vi "Jason Recursion Binary Tube Search SubVI.vi"(6 "Beginning Tube Number":i32, 7 "End Tube Number":i32, 8 "Clear Pin Task In":refnum<k21>, 9 "Write Pin Task In":refnum<k21>, 10 "Sync Pin Task In":refnum<k21>, 11 "Data Pin Task In":refnum<k21>) -> (0 "Clear Pin Task Out":refnum<k21>, 1 "Write Pin Task Out":refnum<k21>, 2 "Sync Pin Task Out":refnum<k21>, 3 "Data Pin Task Out":refnum<k21>)   [LabVIEW 2020]
uses:
  <vilib>/numeric/Random Number (Range) DBL.vi
panel:
  out "Sync Pin Task Out 3":refnum<k21>[](array[refnum])
  out "Write Pin Task Out 3":refnum<k21>[](array[refnum])
  out "Data Pin Task Out 3":refnum<k21>[](array[refnum])
  out "Clear Pin Task Out 3":refnum<k21>[](array[refnum])
  out "Sync Pin Task Out 2":refnum<k21>[](array[refnum])
  out "Write Pin Task Out 2":refnum<k21>[](array[refnum])
  out "Data Pin Task Out 2":refnum<k21>[](array[refnum])
  out "Clear Pin Task Out 2":refnum<k21>[](array[refnum])
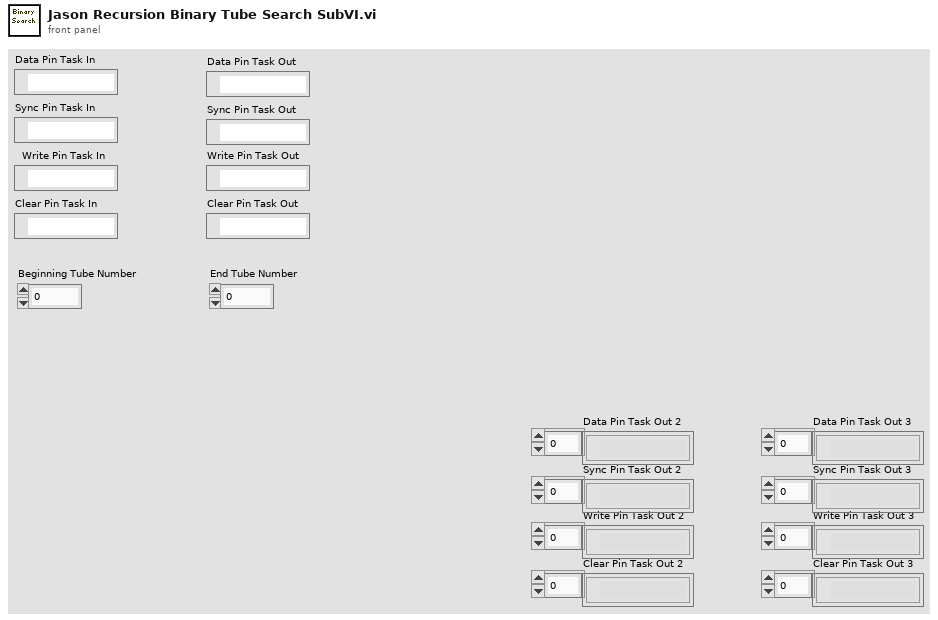
[diagram p1: front panel]
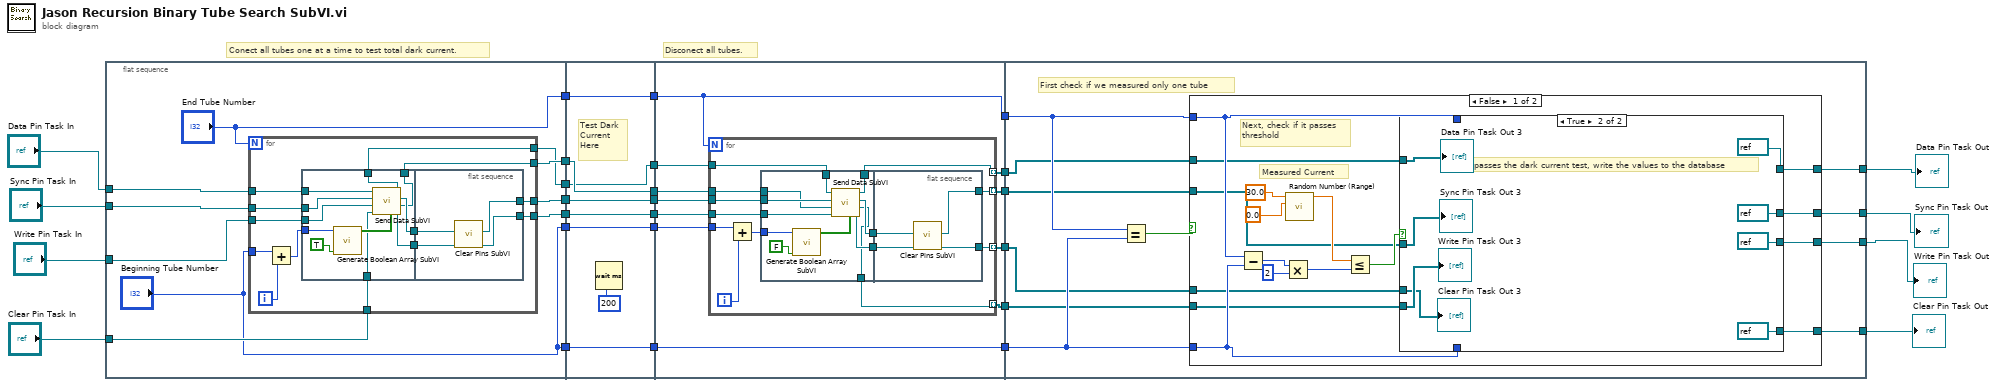
[diagram p0: block diagram]
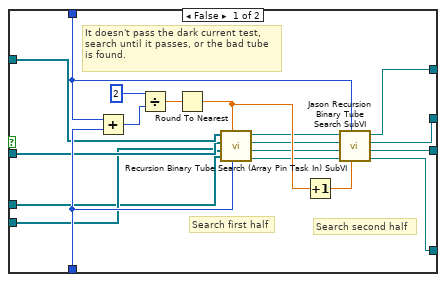
[diagram p2: hidden frame]
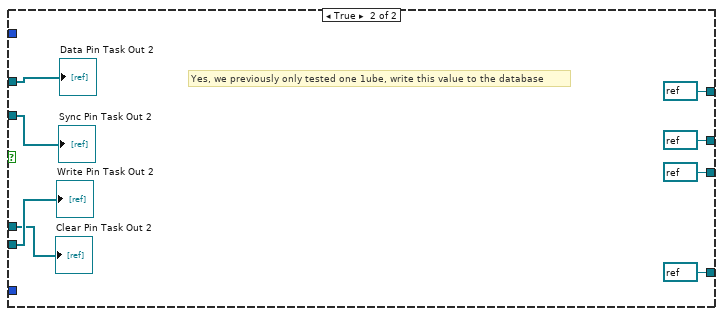
[diagram p3: hidden frame]
diagram:
  # "Disconect all tubes."
  # "Conect all tubes one at a time to test total dark current."
  n1 = flat-sequence {
    tunnel: "Data Pin Task In" -> [w38]
    tunnel: "Sync Pin Task In" -> [w37]
    tunnel: "Write Pin Task In" -> [w36]
    tunnel: "Clear Pin Task In" -> [w35]
    tunnel: ["End Tube Number"] -> w23
    tunnel: [w33] -> w21
    tunnel: [w32] -> w19
    tunnel: [w31] -> w17
    tunnel: [w30] -> w15
    tunnel: ["Beginning Tube Number"] -> w12
    tunnel: ["Beginning Tube Number"] -> w9
    tunnel: [w73] -> w24
    tunnel: w23 -> [w73]
    tunnel: [w72] -> w22
    tunnel: w21 -> [w72]
    tunnel: [w71] -> w20
    tunnel: w19 -> [w71]
    tunnel: [w70] -> w18
    tunnel: w17 -> [w70]
    tunnel: [w69] -> w16
    tunnel: w15 -> [w69]
    tunnel: [w68] -> w13
    tunnel: w12 -> [w68]
    tunnel: [w67] -> w10
    tunnel: w9 -> [w67]
    tunnel: w24 -> [w81]
    tunnel: w22 -> [w85]
    tunnel: w20 -> [w84]
    tunnel: w18 -> [w83]
    tunnel: w16 -> [w82]
    tunnel: [w81] -> w14
    tunnel: w13 -> [w80]
    tunnel: [w79] -> w11
    tunnel: w10 -> [w79]
    tunnel: [w78] -> w8
    tunnel: [w77] -> w7
    tunnel: [w76] -> w6
    tunnel: [w75] -> w5
    tunnel: w14 -> [w123]
    tunnel: w11 -> [w122]
    tunnel: w8 -> [w117]
    tunnel: w7 -> [w116]
    tunnel: w6 -> [w115]
    tunnel: w5 -> [w114]
    tunnel: [w121] -> w4
    tunnel: [w120] -> w3
    tunnel: [w119] -> w2
    tunnel: [w118] -> w1
    frame #0 {
      n2 = for {
        N: "End Tube Number" -> [_]
        tunnel: w38 -> [w51]
        tunnel: w37 -> [w50]
        tunnel: w36 -> [w49]
        tunnel: w35 -> [w48]
        tunnel: [w45] -> w33
        tunnel: [w44] -> w32
        tunnel: [w43] -> w31
        tunnel: [w42] -> w30
        tunnel: "Beginning Tube Number" -> [w39]
        i -> [w40]
        n3 = Add(x=w39, y=w40) -> (x+y=w41:i32)
        n4 = flat-sequence {
          tunnel: w41 -> [w60]
          tunnel: w51 -> [w59]
          tunnel: w50 -> [w58]
          tunnel: w49 -> [w57]
          tunnel: w48 -> [w56]
          tunnel: [w55] -> w47
          tunnel: [w54] -> w46
          tunnel: [w53] -> w43
          tunnel: [w52] -> w42
          tunnel: w47 -> [w66]
          tunnel: w46 -> [w65]
          tunnel: [w64] -> w45
          tunnel: [w63] -> w44
          frame #0 {
            n5 = call "Generate Boolean Array SubVI.vi"("Activate: 1\nDeactivate: 0"=TRUE, "Tube"=w60) -> ("Boolean array"=w61:bool[])  [unwired: 9 in]
            n6 = call "Send Data SubVI.vi"("Data Pin Task In"=w59, "Sync Pin Task In"=w58, "Write Pin Task In"=w57, "Clear Pin Task In"=w56, "Data"=w61) -> ("Data Pin Task Out"=w52:refnum<k21>, "Sync Pin Task Out"=w55:refnum<k21>, "Write Pin Task Out"=w53:refnum<k21>, "Clear Pin Task Out"=w54:refnum<k21>)  [unwired: 1 in]
          }
          frame #1 {
            n7 = call "Clear Pins SubVI.vi"("Clear Pin Task In"=w65, "Sync Pin Task In"=w66) -> ("Clear Pin Task Out"=w63:refnum<k21>, "Sync Pin Task Out"=w64:refnum<k21>)  [unwired: 8 in]
          }
        }
      }
    }
    frame #1 {
      # "Test Dark \nCurrent \nHere"
      n8 = Wait (ms)(milliseconds to wait=u32 200) -> ()  [unwired: 1 out]
    }
    frame #2 {
      n9 = for {
        N: w81 -> [_]
        tunnel: w85 -> [w96]
        tunnel: w84 -> [w95]
        tunnel: w83 -> [w94]
        tunnel: w82 -> [w93]
        tunnel: w80 -> [w90]
        tunnel: [w89] -> w78 mode=indexing
        tunnel: [w88] -> w77 mode=indexing
        tunnel: [w87] -> w76 mode=indexing
        tunnel: [w86] -> w75 mode=indexing
        i -> [w91]
        n10 = Add(x=w90, y=w91) -> (x+y=w92:i32)
        n11 = flat-sequence {
          tunnel: w92 -> [w107]
          tunnel: [w106] -> w98
          tunnel: [w105] -> w97
          tunnel: w96 -> [w104]
          tunnel: w95 -> [w103]
          tunnel: w94 -> [w102]
          tunnel: w93 -> [w101]
          tunnel: [w100] -> w89
          tunnel: [w99] -> w87
          tunnel: w98 -> [w113]
          tunnel: w97 -> [w112]
          tunnel: [w111] -> w88
          tunnel: [w110] -> w86
          frame #0 {
            n12 = call "Generate Boolean Array SubVI.vi"("Activate: 1\nDeactivate: 0"=FALSE, "Tube"=w107) -> ("Boolean array"=w108:bool[])  [unwired: 9 in]
            n13 = call "Send Data SubVI.vi"("Data Pin Task In"=w101, "Sync Pin Task In"=w104, "Write Pin Task In"=w102, "Clear Pin Task In"=w103, "Data"=w108) -> ("Data Pin Task Out"=w100:refnum<k21>, "Sync Pin Task Out"=w106:refnum<k21>, "Write Pin Task Out"=w99:refnum<k21>, "Clear Pin Task Out"=w105:refnum<k21>)  [unwired: 1 in]
          }
          frame #1 {
            n14 = call "Clear Pins SubVI.vi"("Clear Pin Task In"=w112, "Sync Pin Task In"=w113) -> ("Clear Pin Task Out"=w110:refnum<k21>, "Sync Pin Task Out"=w111:refnum<k21>)  [unwired: 8 in]
          }
        }
      }
    }
    frame #3 {
      # "First check if we measured only one tube"
      n15 = Equal?(x=w123, y=w122) -> (x = y?=w124:bool)
      n16 = case shown="False" w124 {
        tunnel: w123 -> [w134 _]
        tunnel: w122 -> [w133 _]
        tunnel: [w132 refnum<k21> refnum ("Data Pin Task Out")] -> w121
        tunnel: [w131 refnum<k21> refnum ("Sync Pin Task Out")] -> w120
        tunnel: [w130 refnum<k21> refnum ("Write Pin Task Out")] -> w119
        tunnel: [w129 refnum<k21> refnum ("Clear Pin Task Out")] -> w118
        tunnel: w117 -> [w128 w172]
        tunnel: w116 -> [w127 w171]
        tunnel: w115 -> [w126 w170]
        tunnel: w114 -> [w125 w169]
        frame False {
          # "Next, check if it passes\nthreshold"
          # "Measured Current"
          n17 = Subtract(x=w134, y=w133) -> (x-y=w136:i32)
          n18 = Multiply(x=w136, y=2) -> (x*y=w141:i32)
          n19 = call-poly <vilib>:"Random Number (Range).vi"("lower bound (0)"=0.0, "upper bound (100)"=30.0) -> ("number"=w140:dbl)  [unwired: 9 in]
          n20 = Less Or Equal?(x=w140, y=w141) -> (x <= y?=w135:bool)
          n21 = case shown="True" w135 {
            tunnel: w134 -> [w157 _]
            tunnel: w133 -> [w150 _]
            tunnel: [w155 refnum<k21> refnum ("Data Pin Task Out")] -> w132
            tunnel: [w154 refnum<k21> refnum ("Sync Pin Task Out")] -> w131
            tunnel: [w153 refnum<k21> refnum ("Write Pin Task Out")] -> w130
            tunnel: [w152 refnum<k21> refnum ("Clear Pin Task Out")] -> w129
            tunnel: w128 -> [w145 w168]
            tunnel: w127 -> [w144 w167]
            tunnel: w126 -> [w143 w166]
            tunnel: w125 -> [w142 w165]
            frame False {
              # "Search second half"
              # "Search first half"
              # "It doesn't pass the dark current test,\nsearch until it passes, or the bad tube\nis found."
              n22 = Add(x=w157, y=w150) -> (x+y=w159:i32)
              n23 = Divide(x=2, y=w159) -> (x/y=w160:dbl)
              n24 = Round To Nearest(number=w160) -> (nearest integer value=w151:dbl)
              n25 = call "Recursion Binary Tube Search (Array Pin Task In) SubVI.vi"("Beginning Tube Number"=w150, "End Tube Number"=w151, "Clear Pin Task In"=w142, "Write Pin Task In"=w143, "Sync Pin Task In"=w144, "Data Pin Task In"=w145) -> ("Clear Pin Task Out"=w146:refnum<k21>, "Write Pin Task Out"=w147:refnum<k21>, "Sync Pin Task Out"=w148:refnum<k21>, "Data Pin Task Out"=w149:refnum<k21>)  [unwired: 2 in]
              n26 = Increment(x=w151) -> (x+1=w156:dbl)
              n27 = call "Jason Recursion Binary Tube Search SubVI.vi"("Beginning Tube Number"=w156, "End Tube Number"=w157, "Clear Pin Task In"=w146, "Write Pin Task In"=w147, "Sync Pin Task In"=w148, "Data Pin Task In"=w149) -> ("Clear Pin Task Out"=w152:refnum<k21>, "Write Pin Task Out"=w153:refnum<k21>, "Sync Pin Task Out"=w154:refnum<k21>, "Data Pin Task Out"=w155:refnum<k21>)  [unwired: 2 in]
            }
            frame True {
              # "It passes the dark current test, write the values to the database"
              "Clear Pin Task Out 3" <- w165
              "Data Pin Task Out 3" <- w168
              "Write Pin Task Out 3" <- w166
              "Sync Pin Task Out 3" <- w167
            }
          }
        }
        frame True {
          # "Yes, we previously only tested one 1ube, write this value to the database"
          "Clear Pin Task Out 2" <- w169
          "Data Pin Task Out 2" <- w172
          "Write Pin Task Out 2" <- w170
          "Sync Pin Task Out 2" <- w171
        }
      }
    }
  }
  "Clear Pin Task Out" <- w1
  "Data Pin Task Out" <- w4
  "Write Pin Task Out" <- w2
  "Sync Pin Task Out" <- w3
